vi "Kundendaten.vi"(8 "error in (no error)":errorcluster) -> (0 "error out":errorcluster)   [LabVIEW 2023]
uses:
  <vilib>/Utility/miscctls.llb/LVRectTypeDef.ctl
panel:
  in  "Numeric":dbl
  in  "Ort":string
  in  "Straße":string
  in  "Firma name":string
  out "Firma":bool
  in  "Blank Button 2":bool
  in  "Blank Button":bool
  in  "Reserve schalter":bool
  in  "Stop Button":bool
  in  "Nachname":string
  in  "Vorname":string
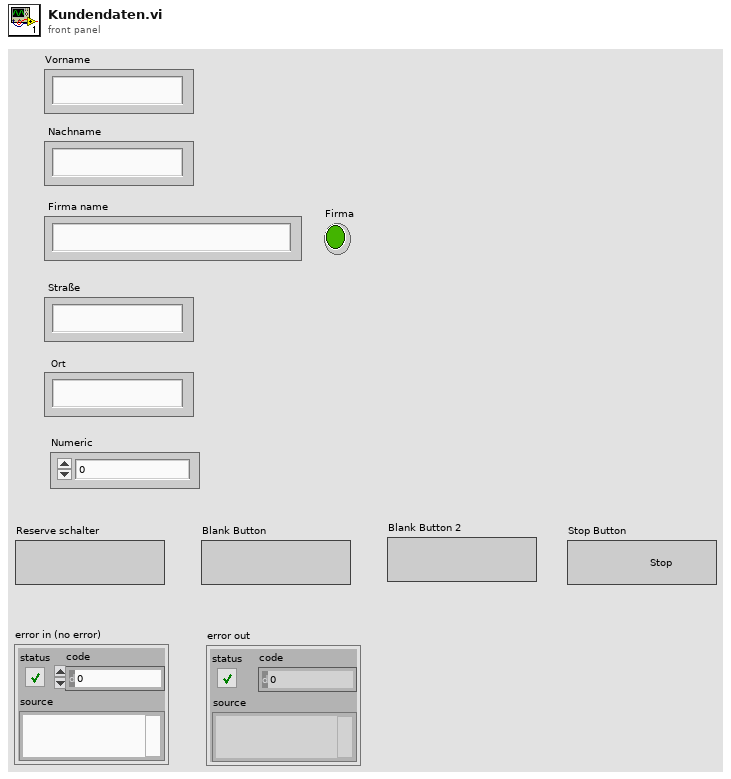
[diagram p1: front panel]
types:
  T1 = typedef "LVRectTypeDef.ctl" = cluster{"Left":i16, "Top":i16, "Right":i16, "Bottom":i16}
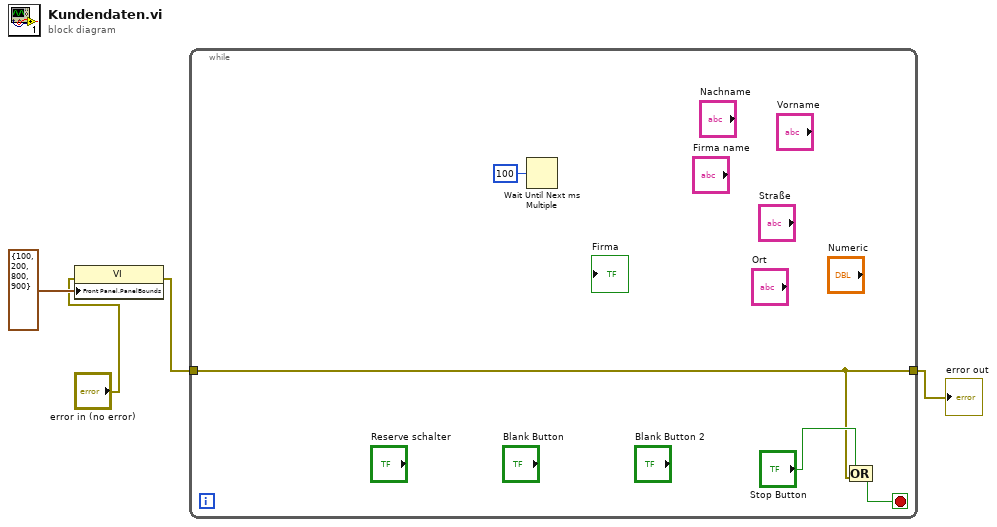
[diagram p0: block diagram]
diagram:
  n1 = property class="VI"(error in="error in (no error)", "Front Panel.PanelBounds"=T1 {"Left"=100, "Top"=200, "Right"=800, "Bottom"=900} ("Front Panel Window:Panel Bounds")) -> (error out=w1:errorcluster)  [unwired: 1 in, 1 out]
  n2 = while {
    tunnel: [w6] -> w4
    tunnel: w1 -> [w6]
    stop <- w7 stop-if-true
    n3 = Wait Until Next ms Multiple(millisecond multiple=u32 100) -> ()  [unwired: 1 out]
    n4 = Compound Arithmetic op=OR("Stop Button", w6) -> (w7:bool)
  }
  "error out" <- w4
